vi "Identify.vi"(8 "error out":errorcluster, 11 "VISA resource name":refnum<visa-resource-name>) -> (0 "error out":errorcluster, 1 "Instrument Firmware Revision":string, 2 "Serial Number":string, 3 "VISA resource name out":refnum<visa-resource-name>, 4 "Device Errors":cluster{"code":i32, "Text":string}[](array[cluster]), 5 "Manufacturer":string, 6 "Model":string, 7 "Instrument identification string":string)   [LabVIEW 2014, in "Stanford Research DG645 - Driver.lvlib"]
doc: "Common IEEE-488.2 Command: *ISDN?\nInstrument Error Check\n\nQuery the instrument identification string. Returns a string similar to 'Stanford Research Systems,DG645,s/n004025,ver1.00.00E'."
uses:
  Stanford Research DG645 - Driver.lvlib
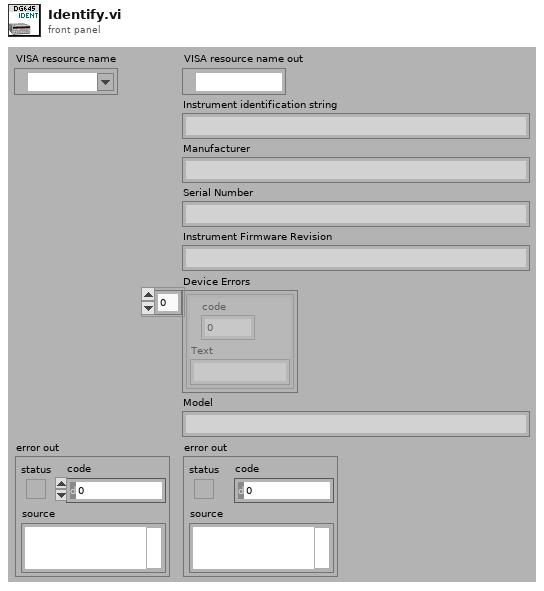
[diagram p1: front panel]
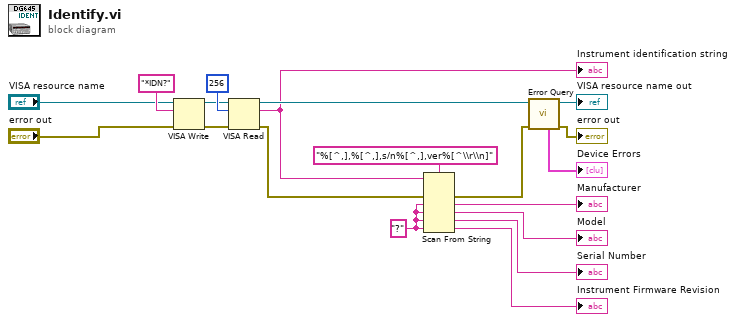
[diagram p0: block diagram]
diagram:
  w8 = "?"
  n1 = VISA Write(VISA resource name="VISA resource name", write buffer="*IDN?" ("ID Query"), error in (no error)="error out") -> (VISA resource name out=w16:refnum<visa-resource-name>, error out=w17:errorcluster)  [unwired: 1 out]
  n2 = VISA Read(VISA resource name=w16, byte count=u32 256, error in (no error)=w17) -> (VISA resource name out=w15:refnum<visa-resource-name>, read buffer=w1:string, error out=w3:errorcluster)  [unwired: 1 out]
  "Instrument identification string" <- w1
  n3 = Scan From String(format string="%[^,],%[^,],s/n%[^,],ver%[^\\r\\n]", input string=w1, error in=w3, default 1=w8, default 2=w8, default 3=w8, default 4=w8) -> (error out=w2:errorcluster, output 1=→"Manufacturer":string, output 2=→"Model":string, output 3=→"Serial Number":string, output 4=→"Instrument Firmware Revision":string)  [unwired: 1 in, 2 out]
  n4 = call "Error Query.vi"("error in (no error)"=w2, "VISA resource name"=w15) -> ("error out"=→"error out":errorcluster, "VISA resource name out"=→"VISA resource name out":refnum<visa-resource-name>, "Device Errors"=→"Device Errors":cluster{"code":i32, "Text":string}[])  [unwired: 7 in]
